vi "Proceed.vi"(7 "component is ready (Y)":bool=TRUE, 8 "error in (no error)":errorcluster, 10 "ProceedMessage":refnum<class "ProceedMessage.lvclass">, 11 "TomoConversion in":refnum<class "TomoConversion.lvclass">) -> (0 "error out":errorcluster, 2 "all observers are ready?":bool, 3 "TomoConversion out":refnum<class "TomoConversion.lvclass">)   [LabVIEW 2012, in "TomoConversion.lvclass"]
uses:
  TomoConversion.lvclass
  <vilib>/Distrio/Murmex/Murmex/Murmex.lvclass
  <userlib>/_OpenG.lib/array/array.llb/Empty 1D Array (String)__ogtk.vi
  <vilib>/Distrio/Murmex/ProceedMessage/ProceedMessage.lvclass
panel:
  # "This method is called when the PROCEED\ntrigger is sent. \n\nOverride this method when your component needs to\nrespond to this trigger. \n\nCall parent for proper implementation"
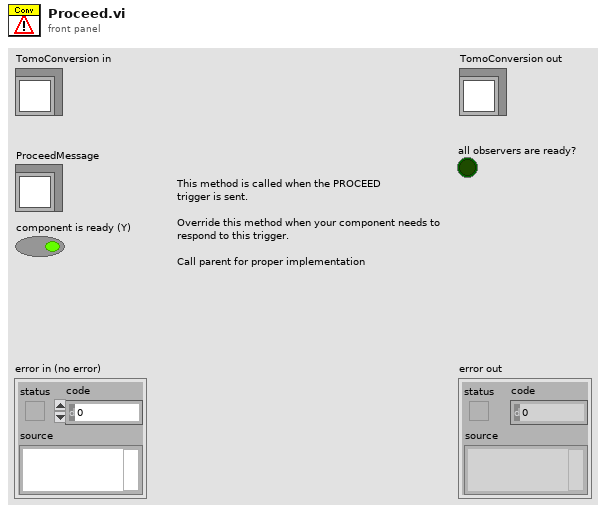
[diagram p1: front panel]
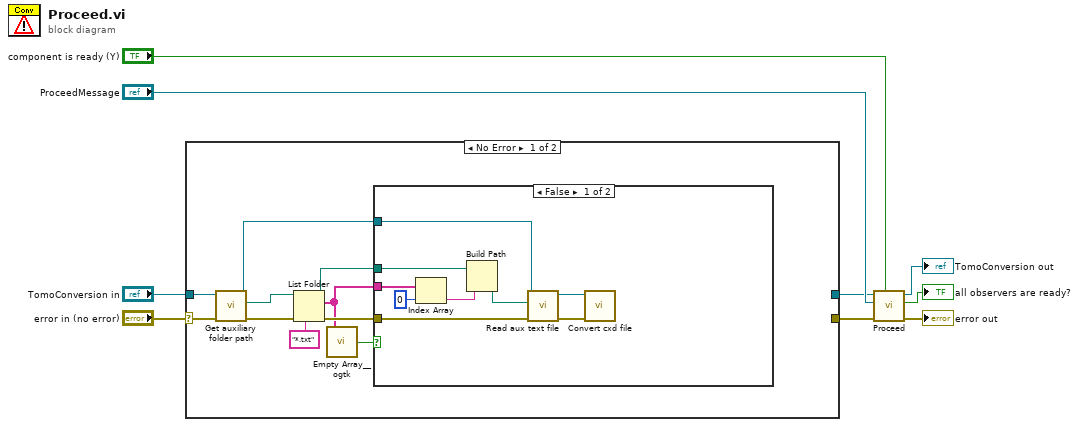
[diagram p0: block diagram]
diagram:
  n1 = case shown="No Error" "error in (no error)" {
    selector: "error in (no error)" -> [w17 w30]
    tunnel: [_ w30] -> w3
    tunnel: [_ w29] -> w2
    tunnel: "TomoConversion in" -> [w18 w29]
    frame No Error {
      n2 = call-dynamic "Get auxiliary folder path.vi"("error in (no error)"=w17, "TomoConversion in"=w18) -> ("error out"=w16:errorcluster, "auxiliary folder path"=w15:path, "TomoConversion out"=w12:refnum<class "TomoConversion.lvclass">)  [unwired: 7 in]
      n3 = List Folder(path=w15, pattern="*.txt", error in=w16) -> (path out=w11:path, filenames=w10:string[], error out=w13:errorcluster)  [unwired: 1 in, 1 out]
      n4 = call-poly <userlib>:"Empty Array__ogtk.vi"("Array"=w10) -> ("Empty Array?"=w14:bool)  [unwired: 8 in]
      n5 = case shown="False" w14 {
        tunnel: w13 -> [w24 _]
        tunnel: w12 -> [w23 _]
        tunnel: w11 -> [w26 _]
        tunnel: w10 -> [w28 _]
        frame False {
          n6 = Index Array(array=w28, index=0) -> (element=w25:string)
          n7 = Build Path(base path=w26, name or relative path=w25) -> (appended path=w22:path)
          n8 = call-dynamic "Read aux text file.vi"("error in (no error)"=w24, "Aux text file path"=w22, "TomoConversion in"=w23) -> ("error out"=w20:errorcluster, "TomoConversion out"=w21:refnum<class "TomoConversion.lvclass">)  [unwired: 7 in]
          n9 = call-dynamic "Convert cxd file.vi"("error in (no error)"=w20, "TomoConversion in"=w21) -> ()  [unwired: 8 in, 2 out]
        }
        frame True {
        }
      }
    }
    frame Error {
    }
  }
  n10 = call-parent "Proceed.vi"("component is ready (Y)"="component is ready (Y)", "error in (no error)"=w3, "ProceedMessage"="ProceedMessage", "Murmex in"=w2) -> ("error out"=→"error out":errorcluster, "all observers are ready?"=→"all observers are ready?":bool, "Murmex out"=→"TomoConversion out":refnum<class "TomoConversion.lvclass">)  [unwired: 5 in]
